vi "Initialize System (Multiple Buses).vi"(0 "bus configuration":T1[](array[typedef]) {"current channels"."physical channels"."channel phase" items=["Phase A (L1)", "Phase B (L2)", "Phase C (L3)", "Phase N (Neutral)"]; "voltage channels"."physical channels"."channel phase" items=["Phase A (L1)", "Phase B (L2)", "Phase C (L3)", "Phase N (Neutral)"]; "symmetrical components calculation" items=["Phase to Phase", "Phase to Neutral"]; "samples per cycle" min=128 max=512}, 11 "error in (no error)":errorcluster) -> (4 "nominal sample rate [Hz]":u16[](array[numeric]), 10 "system info out":refnum<class "EP System Info.lvclass">[](array[class]), 15 "error out":errorcluster)   [LabVIEW 2014, in "NI_EP_Power Quality.lvlib"]
doc: "Sets the basic configuration of the electrical power system based on different line and bus configurations. You must manually select the polymorphic instance you want to use."
uses:
  <vilib>/addons/Electrical Power/PQ/NI_EP_Power Quality.lvlib
  <vilib>/addons/Electrical Power/PQ/Common/Controls/ep_Bus Config.ctl
  <vilib>/addons/Electrical Power/PQ/Common/Controls/ep_Symmetrical Component Calculation.ctl
  <vilib>/addons/Electrical Power/PQ/Common/Controls/ep_Channels Config.ctl
  <vilib>/addons/Electrical Power/PQ/Common/Controls/ep_Channel Phase.ctl
  <vilib>/addons/Electrical Power/PQ/Common/Classes/System Info/EP System Info.lvclass
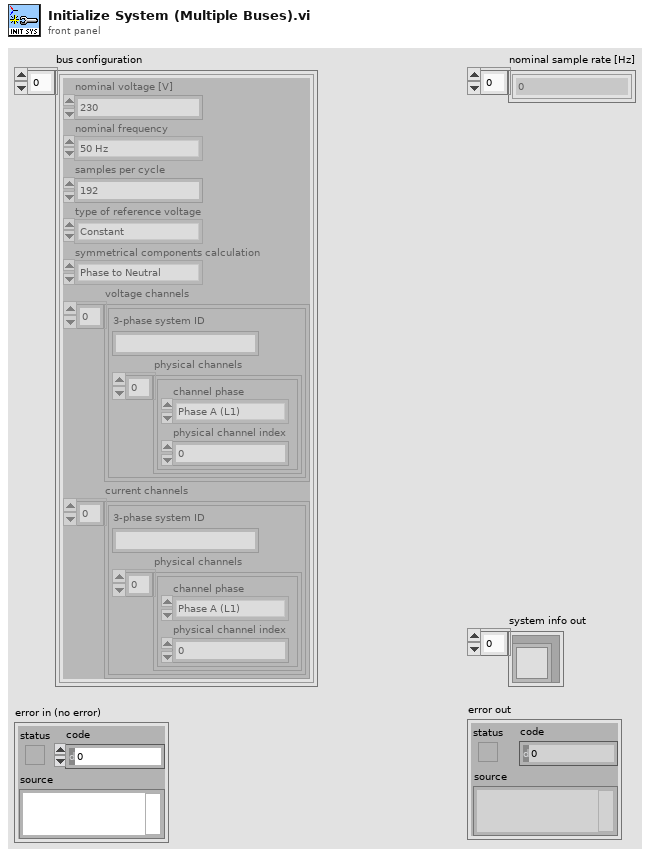
[diagram p1: front panel]
types:
  T1 = typedef "NI_EP_Power Quality.lvlib/ep_Bus Config.ctl" = cluster{"nominal voltage [V]":dbl, "nominal frequency":enum16{"50 Hz", "60 Hz"}, "samples per cycle":u16, "type of reference voltage":enum16{"Constant", "Sliding"}, "symmetrical components calculation":T2, "voltage channels":T3[], "current channels":T3[]}
  T2 = typedef "NI_EP_Power Quality.lvlib/ep_Symmetrical Component Calculation.ctl" = u16
  T3 = typedef "NI_EP_Power Quality.lvlib/ep_Channels Config.ctl" = cluster{"3-phase system ID":string, "physical channels":cluster{"channel phase":T4, "physical channel index":u16}[]}
  T4 = typedef "NI_EP_Power Quality.lvlib/ep_Channel Phase.ctl" = u16
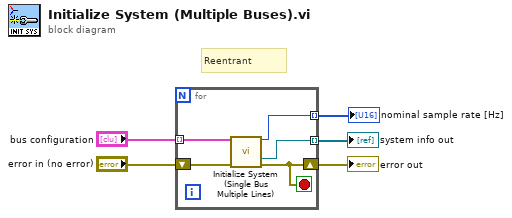
[diagram p0: block diagram]
diagram:
  # "Reentrant"
  n1 = for {
    tunnel: "bus configuration" -> [w9] mode=indexing
    shift-right: [w6] -> w4
    shift-left: "error in (no error)" -> [w10]
    tunnel: [w8] -> w2 mode=indexing
    tunnel: [w7] -> w1 mode=indexing
    stop <- w6 stop-if-true
    n2 = call <vilib>:"Initialize System (Single Bus Multiple Lines).vi"("bus configuration"=w9, "error in (no error)"=w10) -> ("nominal sample rate [Hz]"=w7:u16, "system info out"=w8:refnum<class "EP System Info.lvclass">, "error out"=w6:errorcluster)  [unwired: 11 in]
  }
  "error out" <- w4
  "system info out" <- w2
  "nominal sample rate [Hz]" <- w1
